vi "Cryopump Variable.vi"() -> ()   [LabVIEW 2012]
panel:
  out "Cryopump Array":dbl[](array[numeric])
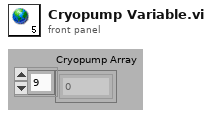
[diagram p1: front panel]
diagram:
